vi "XML 解码.vi"(5 "简易流程Id":u16, 6 "是否是简易流程":bool, 7 "添加的路径":path, 8 "error in (no error)":errorcluster, 11 "参数簇":T1={"启动参数"=1, "启动模式"=enum."跨度核查", "量程"=enum."低量程"} {"启动参数" items=["总磷"=1, "总氮"=2, "氨氮"=3]}) -> (0 "error out":errorcluster, 1 "大小":i32, 2 "步骤文本":u16[](array[numeric]), 3 "步骤详情":u16[](array[numeric]))   [LabVIEW 2016, in "斯坦道氟化物.lvlib"]
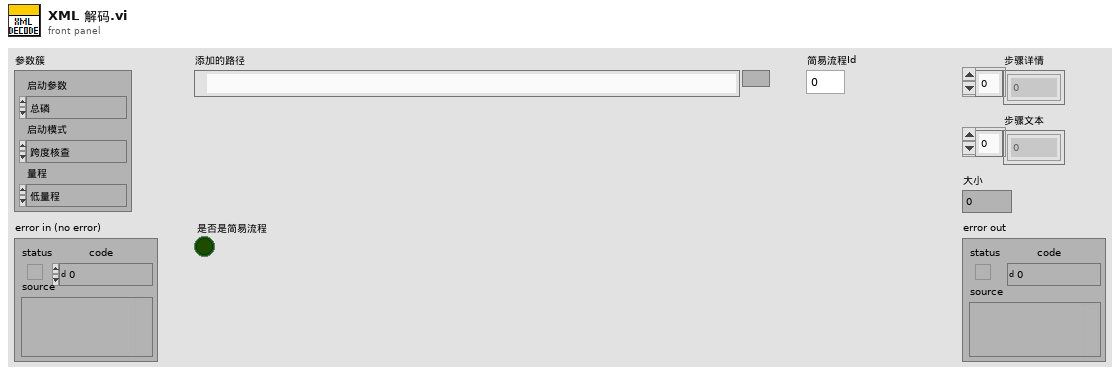
[diagram p1: front panel]
types:
  T1 = cluster{"启动参数":u16, "启动模式":enum16{"跨度核查", "水样测量", "零点核查", "标样核查", "加标回收", "快捷测试", "空白校准", "标样校准"}, "量程":enum16{"低量程", "高量程"}}
  T2 = cluster{"port":i32, "dac":u8, "adc":u8, "time":u16, "步骤名":string}[]
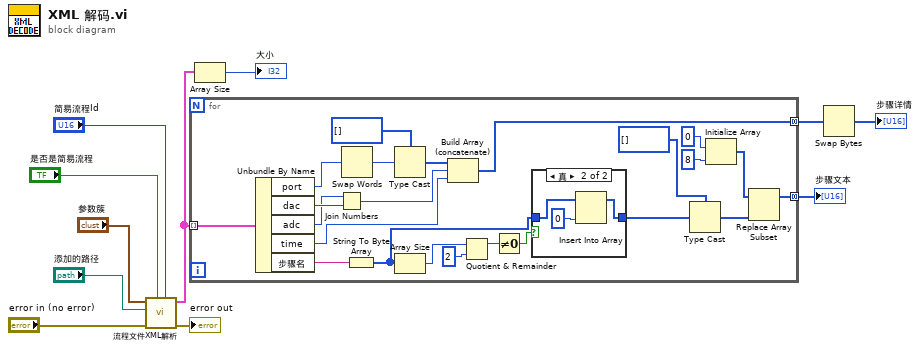
[diagram p0: block diagram]
diagram:
  n1 = call "流程文件XML解析.vi"("简易流程Id"="简易流程Id", "是否是简易流程"="是否是简易流程", "error in (no error)"="error in (no error)", "添加的路径"="添加的路径", "参数簇"="参数簇") -> ("error out"=→"error out":errorcluster, "数组"=w10:T2)  [unwired: 5 in]
  n2 = for {
    tunnel: w10 -> [w34] mode=indexing
    tunnel: [w23] -> w5 mode=concatenating
    tunnel: [w12] -> w6 mode=concatenating
    n3 = Unbundle By Name(w34) -> ("port"=w32:i32, "dac"=w30:u8, "adc"=w29:u8, "time"=w13:u16, "步骤名"=w22:string)
    n4 = Join Numbers(hi=w29, lo=w30) -> ((hi.lo)=w14:u16)
    n5 = Swap Words(1:w32) -> (0:w31:i32)
    n6 = String To Byte Array(string=w22) -> (unsigned byte array=w17:u8[])
    n7 = Type Cast(type=u16[] [], x=w31) -> (*(type *) &x=w15:u16[])
    n8 = Array Size(array=w17) -> (size(s)=w21:i32)
    n9 = Build Array (concatenate)(w15, w14, w13) -> (w12:u16[])
    n10 = Quotient & Remainder(x=w21, y=2) -> (x-y*floor(x/y)=w19:i32)  [unwired: 1 out]
    n11 = Not Equal To 0?(x=w19) -> (x != 0?=w18:bool)
    n12 = case shown="真" w18 {
      tunnel: w17 -> [w35 w38]
      tunnel: [w35 w36] -> w16
      frame False {
      }
      frame True {
        n13 = Insert Into Array(array=w38, new element=u8 0 ("新元素/子数组")) -> (w36:u8[])  [unwired: 1 in]
      }
    }
    n14 = Type Cast(type=u16[] [], x=w16) -> (*(type *) &x=w24:u16[])
    n15 = Initialize Array(u16 0, 8 ("维数大小")) -> (w25:u16[])
    n16 = Replace Array Subset(array=w25, new element=w24) -> (w23:u16[])  [unwired: 1 in]
  }
  "步骤文本" <- w5
  n17 = Array Size(array=w10) -> (size(s)=→"大小":i32)
  n18 = Swap Bytes(anything=w6) -> (byte swapped=→"步骤详情":u16[])
